vi "getActiveSheet.vi"(8 "error in (no error)":errorcluster, 11 "MS-Excel in":refnum<class "MS-Excel.lvclass">) -> (0 "error out":errorcluster, 1 "SheetIndex":i32, 2 "Sheet Ref":refnum<k24>, 3 "MS-Excel out":refnum<class "MS-Excel.lvclass">)   [LabVIEW 2017, in "LabVIEW NPOI.lvlib" / "MS-Excel.lvclass"]
uses:
  MS-Excel.lvclass
  C:/Users/Neo/Desktop/Dev_Tools_BR/LabVIEW_NPOI/lib/NPOI 2.1.1/NPOI.dll
  lib/NPOI 2.1.1/NPOI.dll
  MS-Excel.lvclass/MS-Excel.ctl
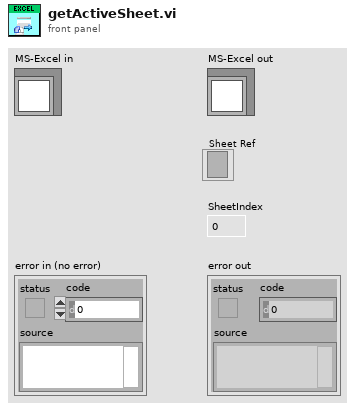
[diagram p1: front panel]
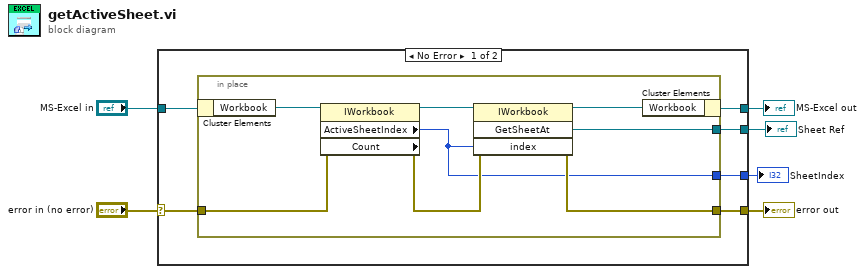
[diagram p0: block diagram]
diagram:
  n1 = case shown="No Error" "error in (no error)" {
    selector: "error in (no error)" -> [w10 w21]
    tunnel: [w9 w21] -> w6
    tunnel: [w12 w22] -> w4
    tunnel: "MS-Excel in" -> [w11 w22]
    tunnel: [w8 _] -> w2
    tunnel: [w7 _] -> w1
    frame No Error {
      n2 = in-place {
        in-place-border: w10 -> [w15]
        in-place-border: [w18] -> w9
        in-place-border: [w17] -> w8
        in-place-border: [w13] -> w7
        n3 = in-place-cluster #1(w11) -> ("Workbook"=w20:refnum<k24>)
        n4 = property class="IWorkbook" props=["ActiveSheetIndex", "Count"](reference=w20, error in=w15) -> (reference out=w16:refnum<k24>, error out=w14:errorcluster, "ActiveSheetIndex"=w13:i32)  [unwired: 1 out]
        n5 = invoke class="IWorkbook" method="GetSheetAt"(reference=w16, error in=w14, "index"=w13) -> (reference out=w19:refnum<k24>, error out=w18:errorcluster, "GetSheetAt"=w17:refnum<k24>)  [unwired: 1 in, 1 out]
        n6 = in-place-cluster #1("Workbook"=w19) -> (w12:refnum<class "MS-Excel.lvclass">)
      }
    }
    frame Error {
    }
  }
  "error out" <- w6
  "MS-Excel out" <- w4
  "Sheet Ref" <- w2
  "SheetIndex" <- w1
